vi "Stop Core.vi"(10 "final error code":i32, 11 "Actor in":refnum<class "Actor.lvclass">) -> (3 "Actor out":refnum<class "Actor.lvclass">)   [LabVIEW 2020, in "Actor Framework.lvlib" / "Actor.lvclass"]
doc: "<p>(<strong>Filename</strong>: <span class=\"dnl\">Actor Framework.lvlib:Actor.lvclass:Stop Core.vi</span>)</p>\n<p>Defines what the actor does before it stops. Use the <strong>final error code</strong> input to determine whether the actor shut down in response to an error.</p>\n<p>By default, this method passes the Stop message along to all <a href=\"nihelplauncher://docs/csh?context=lvcore_lvcomm_af_launch_nested_actor\">auto-stop nested actors</a>. A descendant class may override this method to define additional behavior, such as shutting down any processes the actor initiated in its override of the <a href=\"nihelplauncher://docs/csh?context=lvcore_lvcomm_af_actor_core\">Actor Core</a> method.</p>"
uses:
  Actor.lvclass
  Actor.lvclass/Actor.ctl
  Message Enqueuer/Message Enqueuer.lvclass
  Stop Msg/Stop Msg.lvclass/Stop Msg.ctl
  Message Enqueuer/Message Enqueuer.lvclass/Message Enqueuer.ctl
  Stop Msg/Send Emergency Stop.vi
  Stop Msg/Send Normal Stop.vi
  Message Enqueuer/Enqueue Critical.vi
  Message Enqueuer/Enqueue.vi
  Stop Msg/Stop Msg.lvclass
  C:/justACS/Actor Framework/Core/ActorFramework/Message/Message.lvclass
  <vilib>/Utility/LVClass/Get LV Class Name.vi
  tracing/Trace Generation/Generate Trace for Message.vi
  Message Priority Queue/Priority Enqueue.vi
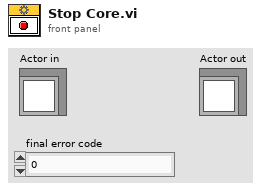
[diagram p1: front panel]
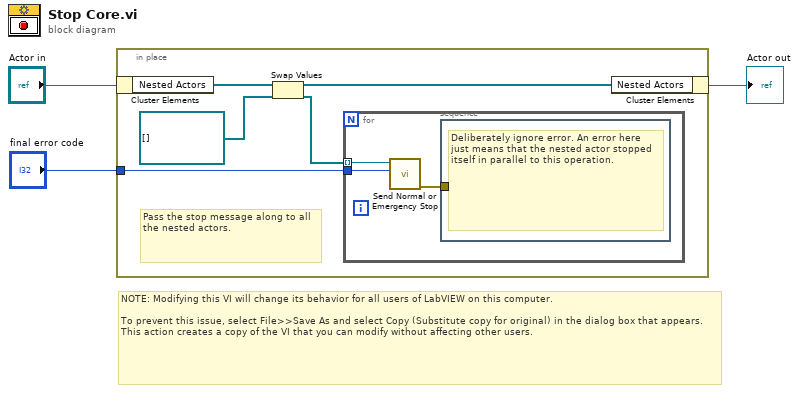
[diagram p0: block diagram]
diagram:
  # "NOTE: Modifying this VI will change its behavior for all users of LabVIEW on this computer.\n\nTo prevent this issue, select File>>Save As and select Copy (Substitute copy for original) in the dialog box that appears. This action creates a copy of the VI that you can modify without affecting other users."
  n1 = in-place {
    in-place-border: "final error code" -> [w4]
    # "Pass the stop message along to all the nested actors."
    n2 = in-place-cluster #1("Actor in") -> ("Nested Actors"=w8:refnum<class "Message Enqueuer.lvclass">[])
    n3 = Swap Values(12:w8, 14:refnum<class "Message Enqueuer.lvclass">[] [] ("Nested Actors")) -> (1:w6:refnum<class "Message Enqueuer.lvclass">[], 3:w5:refnum<class "Message Enqueuer.lvclass">[])  [unwired: 1 in]
    n4 = for {
      tunnel: w5 -> [w11] mode=indexing
      tunnel: w4 -> [w10]
      n5 = call "Send Normal or Emergency Stop.vi"("final error code"=w10, "Message Enqueuer"=w11) -> ("error out"=w9:errorcluster)  [unwired: 9 in]
      n6 = stacked-sequence {
        tunnel: w9 -> [_]
        frame #0 {
          # "Deliberately ignore error. An error here just means that the nested actor stopped itself in parallel to this operation."
        }
      }
    }
    n7 = in-place-cluster #1("Nested Actors"=w6) -> (→"Actor out":refnum<class "Actor.lvclass">)
  }
